vi "_srcipt_text_replace.vi"(6 "スクリプトパス":path=path "G:/fujii/Band10/Labview_ALMA/MIX10/Mixスクリプト", 8 "バッファ":string="Control\nTh, 299.000000\nTc, 83.000000\nDataパス, G:\\assembly\\SN02\\CCA02-11\\111229_DSB_EQ\nHOT/COLD,1\nMPIoffset,23.144000\n\nBias_Lo_equip\nWCA LO YTO Low, 14.650000\nWCA LO YTO High 17.500000\n \nCAN node\nProgram running.\nDo not turn off power to CAN nodes.\n\r\rCAN node with adress x13 found at Node index 00\rS/N: 10 CA E5 4B 01 08 00 0A\r----------\r\r\nAMBSI CAN Library V1.1.2\r\nAMBSI Firmware V1.0.1\r\nFEMC Firmware V2.5.0\r\nFPGA V2.1.0\r\n10 61 15 E4 1 8 0 3B\r\n1 C2 44 A0 13 0 0 3D\r\n1 62 12 81 14 0 0 ED\r\n1 B3 3A 4F 14 0 0 F4\r\n23 90 3C E9 0 0 0 66\r\n0 0 0 0 0 0 0 0\r\n\n\nscript file\n_cart_dsb_post.txt", 9 "Bias_LO_equip":T1={"Node address"=19, "CAN Interface"="CAN0", "Cartridge band"=10, "Slave Node in"={"Address"=19, "Serial Number"=[16, -54, -27, 75, 1, 8, 0, 10]}, "ObjHandle out"=18, "POL"=0, "sb"=1, "GPIB_SM (SIS S,V)"="24", "GPIB_DMM (SIS I)"="22", "GPIB_SM (MAG I) "="25", "GPIB_SG(LO)"="19", "GPIB_PW (PAMP) "="6", "GPIB_TMP1(8ch)"="12", "GPIB_TMP2(2ch)  "="13", "WCA_avg"=10, "Rsen"=10.0, "BiasModule"=1, "LOModule "=2, "WCA_LO_FREQ_SET"={"YTO Low freq. [GHz]"=14.65, "YTO High freq. [GHz]"=17.5, "Kvco"=1, "Lock Pol."=0, "SET LO FREQ"=97.111115, "Multiplier"=6.0, "YTO (HEX)"=2196, "YTO ( FREQ)"=16.178352, "NULL PLL INTEGRATOR"=FALSE}, "Res for"=0} {"Res for" items=["none", "series res", "parallel res"]; "WCA_LO_FREQ_SET"."YTO ( FREQ)" min=25 max=150 step=0.0001 format="%.3f"; "WCA_LO_FREQ_SET"."Multiplier" min=3 max=6 step=3; "WCA_LO_FREQ_SET"."SET LO FREQ" min=25 max=150 step=0.0001 format="%.3f"; "WCA_LO_FREQ_SET"."Lock Pol." items=["Lower", "Upper"]; "WCA_LO_FREQ_SET"."Kvco" items=["7.5MHz/V", "15MHz/V"]; "WCA_LO_FREQ_SET"."YTO High freq. [GHz]" format="%.3f"; "WCA_LO_FREQ_SET"."YTO Low freq. [GHz]" format="%.3f"; "BiasModule" items=["B10Lab Bias"=0, "WCA BiasModule"=1, "none"=99]; "Slave Node in"."Serial Number" format="%.0x"; "Slave Node in"."Address" format="%.0x"; "Cartridge band" max=10 step=1; "Node address" format="%.0x"}, 10 "Control":T2={"GPIB_ATT"="28", "6501Dev#"=1, "GPIB_SP"="18", "GPIB_PM"="13", "GPIB_DSA"="11", "GPIB_DMM (TPD)"="23", "MPI COM"="COM10", "mortor設定"=[{"Axis"=0, "ID"=0, "HIspeed"=200.0, "LOspeed"=100.0, "ACCEL(ms)"=100.0, "Sratio"=50.0, "フリーラン\n"=FALSE, "文字列"="DSB HOT/COLD"}, {"Axis"=1, "ID"=0, "HIspeed"=4.0, "LOspeed"=4.0, "ACCEL(ms)"=100.0, "Sratio"=50.0, "フリーラン\n"=TRUE, "文字列"="SubMM Att"}, {"Axis"=0, "ID"=0, "HIspeed"=200.0, "LOspeed"=100.0, "ACCEL(ms)"=100.0, "Sratio"=50.0, "フリーラン\n"=FALSE, "文字列"="MPI Port1"}, {"Axis"=1, "ID"=0, "HIspeed"=200.0, "LOspeed"=100.0, "ACCEL(ms)"=100.0, "Sratio"=50.0, "フリーラン\n"=FALSE, "文字列"="MPI Port2"}, {"Axis"=1, "ID"=0, "HIspeed"=200.0, "LOspeed"=100.0, "ACCEL(ms)"=100.0, "Sratio"=50.0, "フリーラン\n"=TRUE, "文字列"="gainComp"}], "DATAパス"=path "G:/assembly/SN02/CCA02-11/111229_DSB_EQ", "mixer param file "=path "C:/Documents and Settings/band10/デスクトップ/data/cartridge/SN06/CCA06-11_mixerparam.csv", "comment"="111229_CCA02-11EQ_DSB", "Cartridge SN"="003601", "Th"=299.0, "Tc"=83.0, "Set_SIS_volt"=2.25, "Offset"=0.0, "control"=0, "FreqLO"=874.0, "Set_Mag_Cur"=9.7, "MPI offset(mm)"=23.144, "HOT/COLD"=1} {"HOT/COLD" items=["DSB", "SBR (Cart.)"]; "control" items=["CLOSE LOOP", "OPEN LOOP", "Not Control"]}, 11 "input":string) -> (3 "output":string)   [LabVIEW 2017]
panel:
  # "LO freq. [GHz]"
  # "YTO LOW\n/High Freq."
  # "ZERO Intgrtr"
  # "Node Address"
  # "Serial Number"
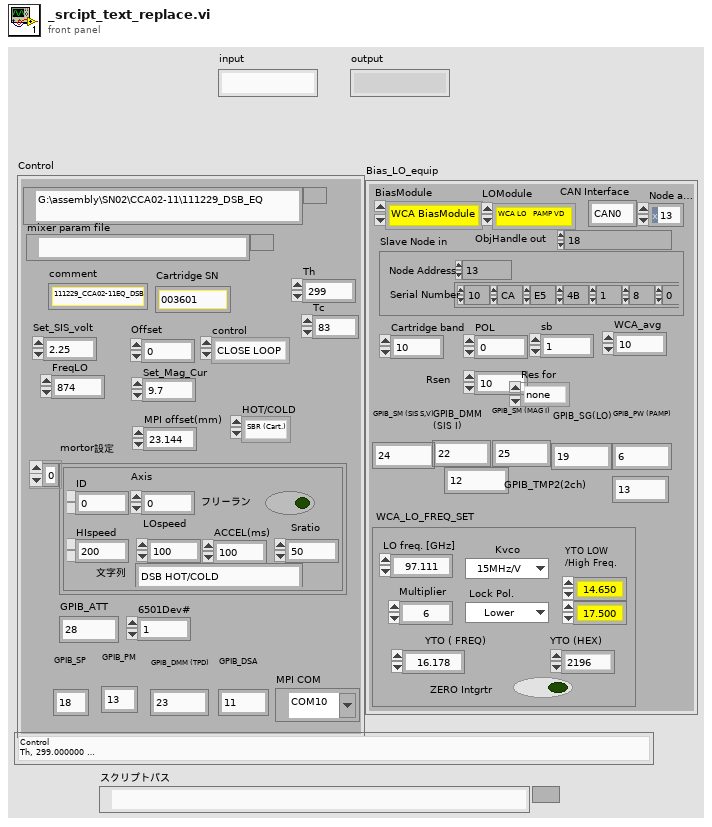
[diagram p1: front panel]
types:
  T1 = cluster{"Node address":u16, "CAN Interface":string, "Cartridge band":u32, "Slave Node in":cluster{"Address":i16, "Serial Number":i8[]}, "ObjHandle out":u32, "POL":u32, "sb":u32, "GPIB_SM (SIS S,V)":string, "GPIB_DMM (SIS I)":string, "GPIB_SM (MAG I) ":string, "GPIB_SG(LO)":string, "GPIB_PW (PAMP) ":string, "GPIB_TMP1(8ch)":string, "GPIB_TMP2(2ch)  ":string, "WCA_avg":i32, "Rsen":dbl, "BiasModule":u16, "LOModule ":u16, "WCA_LO_FREQ_SET":cluster{"YTO Low freq. [GHz]":sgl, "YTO High freq. [GHz]":sgl, "Kvco":u16, "Lock Pol.":u16, "SET LO FREQ":sgl, "Multiplier":sgl, "YTO (HEX)":u16, "YTO ( FREQ)":sgl, "NULL PLL INTEGRATOR":bool}, "Res for":u16}
  T2 = cluster{"GPIB_ATT":string, "6501Dev#":i16, "GPIB_SP":string, "GPIB_PM":string, "GPIB_DSA":string, "GPIB_DMM (TPD)":string, "MPI COM":refnum<visa-resource-name>, "mortor設定":cluster{"Axis":i16, "ID":i16, "HIspeed":dbl, "LOspeed":dbl, "ACCEL(ms)":dbl, "Sratio":dbl, "フリーラン\n":bool, "文字列":string}[], "DATAパス":path, "mixer param file ":path, "comment":string, "Cartridge SN":string, "Th":dbl, "Tc":dbl, "Set_SIS_volt":dbl, "Offset":dbl, "control":u16, "FreqLO":dbl, "Set_Mag_Cur":dbl, "MPI offset(mm)":dbl, "HOT/COLD":u16}
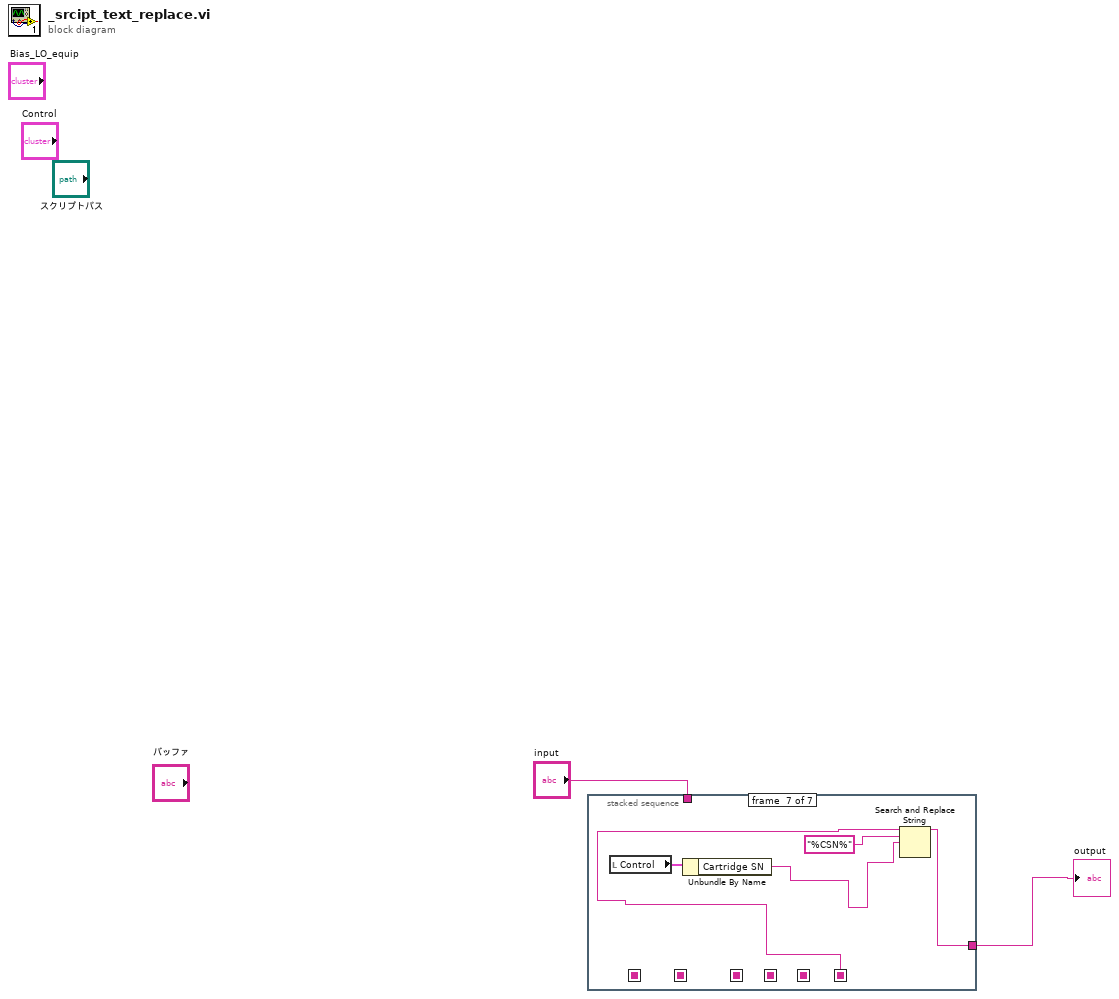
[diagram p0: block diagram]
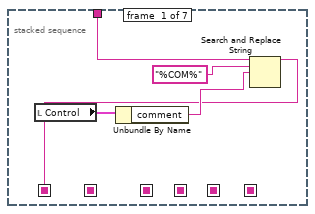
[diagram p2: hidden frame]
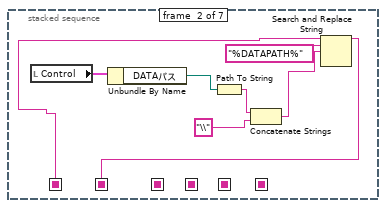
[diagram p3: hidden frame]
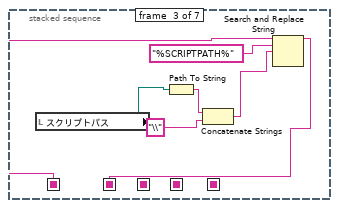
[diagram p4: hidden frame]
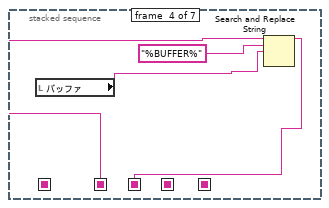
[diagram p5: hidden frame]
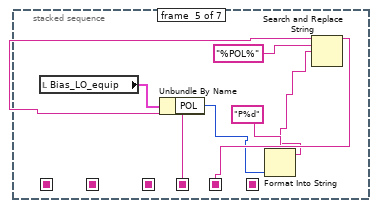
[diagram p6: hidden frame]
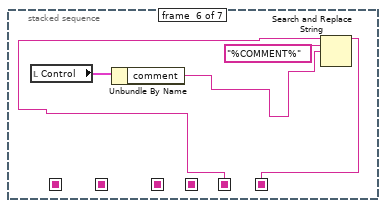
[diagram p7: hidden frame]
diagram:
  n1 = stacked-sequence {
    seq-local: [w3 _ _ _ _ _ _] -> [_ w9 _ _ _ _ _]
    seq-local: [_ w8 _ _ _ _ _] -> [_ _ w18 _ _ _ _]
    seq-local: [_ _ w16 _ _ _ _] -> [_ _ _ w24 _ _ _]
    seq-local: [_ _ _ w23 _ _ _] -> [_ _ _ _ w32 _ _]
    seq-local: [_ _ _ _ w31 _ _] -> [_ _ _ _ _ w35 _]
    seq-local: [_ _ _ _ _ w34 _] -> [_ _ _ _ _ _ w40]
    tunnel: "input" -> [w4 _ _ _ _ _ _]
    tunnel: [_ _ _ _ _ _ w39] -> w1
    frame #0 {
      n2 = local read "Control"() -> (w6:T2)
      n3 = Unbundle By Name(w6) -> ("comment"=w5:string)
      n4 = Search and Replace String(input string=w4, search string="%COM%", replace string=w5) -> (result string=w3:string)  [unwired: 5 in, 3 out]
    }
    frame #1 {
      n5 = local read "Control"() -> (w10:T2)
      n6 = Unbundle By Name(w10) -> ("DATAパス"=w12:path)
      n7 = Path To String(path=w12) -> (string=w13:string)
      n8 = Concatenate Strings(w13, "\\") -> (w15:string)
      n9 = Search and Replace String(input string=w9, search string="%DATAPATH%", replace string=w15) -> (result string=w8:string)  [unwired: 5 in, 3 out]
    }
    frame #2 {
      n10 = local read "スクリプトパス"() -> (w17:path)
      n11 = Path To String(path=w17) -> (string=w20:string)
      n12 = Concatenate Strings(w20, "\\") -> (w22:string)
      n13 = Search and Replace String(input string=w18, search string="%SCRIPTPATH%", replace string=w22) -> (result string=w16:string)  [unwired: 5 in, 3 out]
    }
    frame #3 {
      n14 = local read "バッファ"() -> (w25:string)
      n15 = Search and Replace String(input string=w24, search string="%BUFFER%", replace string=w25) -> (result string=w23:string)  [unwired: 5 in, 3 out]
    }
    frame #4 {
      n16 = local read "Bias_LO_equip"() -> (w27:T1)
      n17 = Unbundle By Name(w27) -> ("POL"=w29:u32)
      n18 = Format Into String(format string="P%d", w29) -> (resulting string=w28:string)  [unwired: 2 in, 1 out]
      n19 = Search and Replace String(input string=w32, search string="%POL%", replace string=w28) -> (result string=w31:string)  [unwired: 5 in, 3 out]
    }
    frame #5 {
      n20 = local read "Control"() -> (w37:T2)
      n21 = Unbundle By Name(w37) -> ("comment"=w36:string)
      n22 = Search and Replace String(input string=w35, search string="%COMMENT%", replace string=w36) -> (result string=w34:string)  [unwired: 5 in, 3 out]
    }
    frame #6 {
      n23 = local read "Control"() -> (w42:T2)
      n24 = Unbundle By Name(w42) -> ("Cartridge SN"=w41:string)
      n25 = Search and Replace String(input string=w40, search string="%CSN%", replace string=w41) -> (result string=w39:string)  [unwired: 5 in, 3 out]
    }
  }
  "output" <- w1
